vi "Configure Current Limit.vi"(8 "error in (no error)":errorcluster, 10 "Current Limit (A)":dbl=0.04 format="%#_13p", 11 "SSC":T1[](array[typedef])) -> (0 "error out":errorcluster, 3 "DCPower SSC out":T1[](array[typedef]))   [LabVIEW 2019]
uses:
  Instrument Control/DCPower/SSC DCPower/SSC DCPower.ctl
  <instrlib>/niDCPower/nidcpower.llb/niDCPower Source Mode.ctl
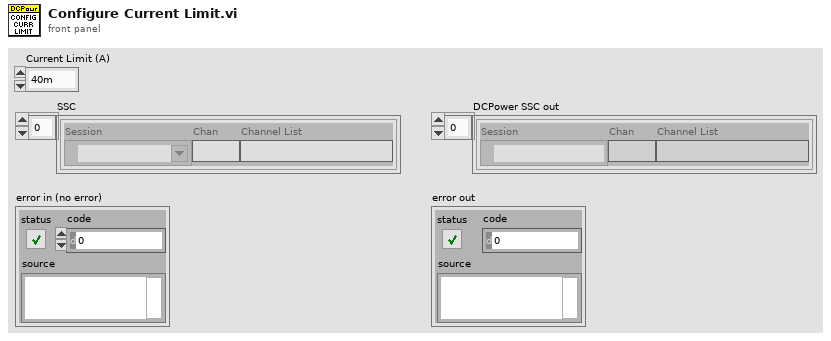
[diagram p1: front panel]
types:
  T1 = typedef "SSC DCPower.ctl" = cluster{"Session":refnum<k15>, "Chan":string, "Channel List":string}
  T2 = typedef "niDCPower Source Mode.ctl" = i32
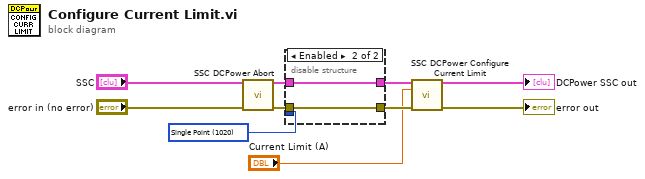
[diagram p0: block diagram]
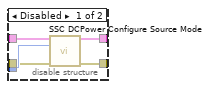
[diagram p2: hidden frame]
diagram:
  w10 = T2 1020 items=["Single Point"=1020, "Sequence"=1021] ("Source Mode")
  n1 = call "SSC DCPower Abort.vi"("DCPower SSC in"="SSC", "error in"="error in (no error)") -> ("DCPower SSC out"=w2:T1[], "error out"=w7:errorcluster)  [unwired: 12 in]
  n2 = disable-structure shown="Enabled" {
    disable-tunnel: w10 -> [w15 _]
    disable-tunnel: [w14 w16] -> w9
    disable-tunnel: w7 -> [w13 w16]
    disable-tunnel: w2 -> [w12 w17]
    disable-tunnel: [w11 w17] -> w1
    frame Disabled {
      n3 = call "SSC DCPower Configure Source Mode.vi"("DCPower SSC in"=w12, "Source Mode"=w15, "error in"=w13) -> ("DCPower SSC out"=w11:T1[], "error out"=w14:errorcluster)  [unwired: 11 in]
    }
    frame Enabled {
    }
  }
  n4 = call "SSC DCPower Configure Current Limit.vi"("DCPower SSC in"=w1, "Current Limit (A)"="Current Limit (A)", "error in"=w9) -> ("DCPower SSC out"=→"DCPower SSC out":T1[], "error out"=→"error out":errorcluster)  [unwired: 11 in]
